vi "FTW-Actor-QueryConfigurationParameter.vi"(0 "FTW Actor":refnum<class "FTW-Actor.lvclass">, 5 "Config Parameter (Type and Default)":string, 11 "error in":errorcluster) -> (4 "FTW Actor out":refnum<class "FTW-Actor.lvclass">, 6 "Value":string, 15 "error out":errorcluster)   [LabVIEW 2012, in "FTW-Actor.lvclass"]
uses:
  FTW-Actor.lvclass
  Container/FTW-Container.lvclass
panel:
  # "Inputs"
  # "Outputs"
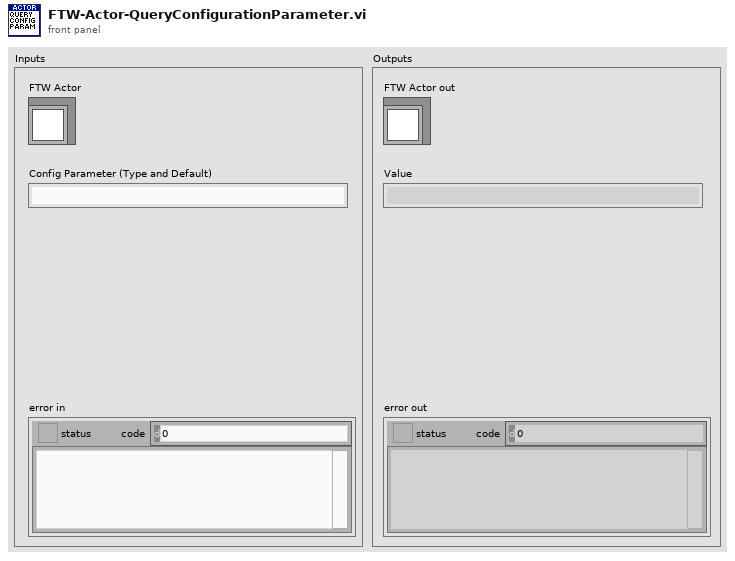
[diagram p1: front panel]
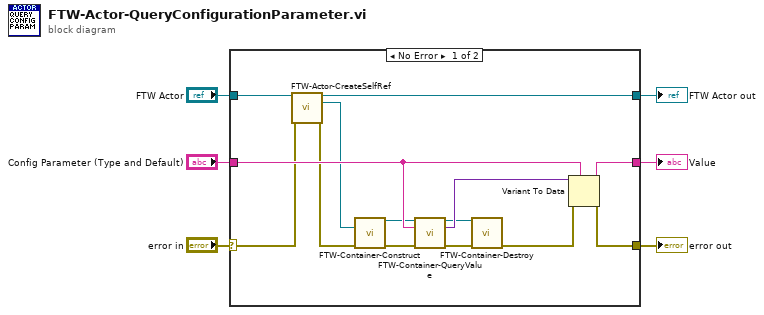
[diagram p0: block diagram]
diagram:
  n1 = case shown="No Error" "error in" {
    selector: "error in" -> [w14 w21]
    tunnel: [w20 w21] -> w6
    tunnel: "FTW Actor" -> [w16 w23]
    tunnel: [w15 w23] -> w4
    tunnel: "Config Parameter (Type and Default)" -> [w19 w22]
    tunnel: [w18 w22] -> w2
    frame No Error {
      n2 = call "FTW-Actor-CreateSelfRef.vi"("FTW Actor"=w16, "error in"=w14) -> ("FTW Actor out"=w15:refnum<class "FTW-Actor.lvclass">, "Reference to Self"=w13:refnum<class "FTW-ActorReference.lvclass">, "error out"=w10:errorcluster)  [unwired: 11 in]
      n3 = call "FTW-Container-Construct.vi"("LabVIEW Data Structure"=w13, "error in"=w10) -> ("Container"=w12:refnum<class "FTW-Container.lvclass">, "error out"=w11:errorcluster)  [unwired: 12 in]
      n4 = call "FTW-Container-QueryValue.vi"("Container"=w12, "Type and Defaults"=w19, "error in"=w11) -> ("Container out"=w9:refnum<class "FTW-Container.lvclass">, "Result"=w17:variant, "error out"=w8:errorcluster)  [unwired: 10 in]
      n5 = call "FTW-Container-Destroy.vi"("Container"=w9, "error in"=w8) -> ("error out"=w7:errorcluster)  [unwired: 13 in]
      n6 = Variant To Data(error in=w7, type=w19, Variant=w17) -> (data=w18:string, error out=w20:errorcluster)
    }
    frame Error {
    }
  }
  "error out" <- w6
  "FTW Actor out" <- w4
  "Value" <- w2
